vi "Get_Files_in_Directory.vi"(0 "File_Names_In":string[](array[string]), 5 "File_Path":path, 7 "First_Call":bool, 11 "Error_In":errorcluster) -> (4 "File_Names_Out":string[](array[string]), 15 "Error_Out":errorcluster)   [LabVIEW 2021]
doc: "Used to get the Files in the Directory."
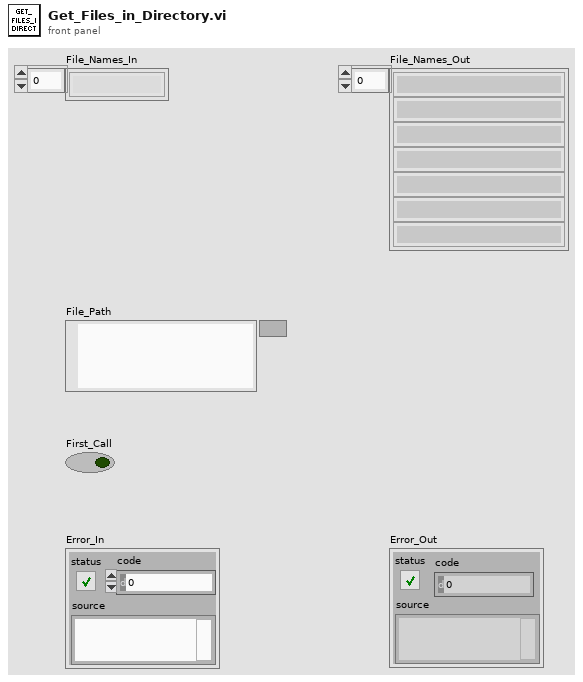
[diagram p1: front panel]
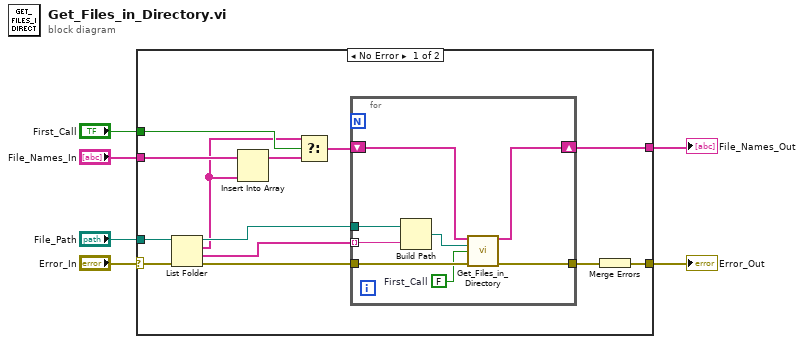
[diagram p0: block diagram]
diagram:
  n1 = case shown="No Error" "Error_In" {
    selector: "Error_In" -> [w16 w29]
    tunnel: "File_Names_In" -> [w9 w28]
    tunnel: [w17 w29] -> w5
    tunnel: "File_Path" -> [w14 _]
    tunnel: [w12 w28] -> w2
    tunnel: "First_Call" -> [w10 _]
    frame No Error {
      n2 = List Folder(path=w14, error in=w16) -> (path out=w13:path, filenames=w8:string[], folder names=w15:string[], error out=w18:errorcluster)  [unwired: 2 in]
      n3 = Insert Into Array(array=w9, new element=w8) -> (w7:string[])  [unwired: 1 in]
      n4 = Select(t=w8, s=w10, f=w7) -> (s? t:f=w11:string[])
      n5 = for {
        tunnel: w15 -> [w24] mode=indexing
        tunnel: w13 -> [w23]
        tunnel: w18 -> [w26]
        tunnel: [w27] -> w19
        shift-right: [w21] -> w12
        shift-left: w11 -> [w25]
        w20 = FALSE  # First_Call
        n6 = Build Path(base path=w23, name or relative path=w24) -> (appended path=w22:path)
        n7 = call "Get_Files_in_Directory.vi"("File_Names_In"=w25, "File_Path"=w22, "First_Call"=w20, "Error_In"=w26) -> ("File_Names_Out"=w21:string[], "Error_Out"=w27:errorcluster)  [unwired: 10 in]
      }
      n8 = Merge Errors(w19) -> (w17:errorcluster)
    }
    frame Error {
    }
  }
  "Error_Out" <- w5
  "File_Names_Out" <- w2
